vi "Vision Global.vi"() -> ()   [LabVIEW 2015]
uses:
  Camera Settings Type Def.ctl
  <vilib>/Rock Robotics/WPI/Camera/WPI_CameraWhite Balance Values.ctl
  <vilib>/Rock Robotics/WPI/Camera/WPI_CameraExposure Values.ctl
panel:
  out "Update Camera Settings":bool
  in  "Camera Settings":T1={"FPS"=0.0, "White Balance"=enum."Fixed indoor", "Exposure"=enum."Flicker-free 60 Hz", "Compression"=0.0, "Brightness"=0.0}
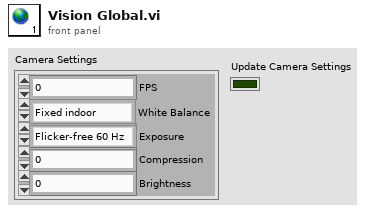
[diagram p1: front panel]
types:
  T1 = typedef "Camera Settings Type Def.ctl" = cluster{"FPS":dbl, "White Balance":T2, "Exposure":T3, "Compression":dbl, "Brightness":dbl}
  T2 = typedef "WPI_CameraWhite Balance Values.ctl" = enum16{"Auto", "Fixed indoor", "Fixed outdoor 1", "Fixed outdoor 2", "Fixed fluorescent 1", "Fixed fluorescent 2", "Hold current", "Custom"}
  T3 = typedef "WPI_CameraExposure Values.ctl" = enum16{"Auto", "Flicker-free 50 Hz", "Flicker-free 60 Hz", "Hold current", "Custom"}
diagram:
